vi "Continuous SFM Test.vi"() -> ()   [LabVIEW 2015]
uses:
  Waveform VIs/FM Sweep VIs/SFM-Params.ctl
panel:
  out "Waveform Graph":dbl[](graph)
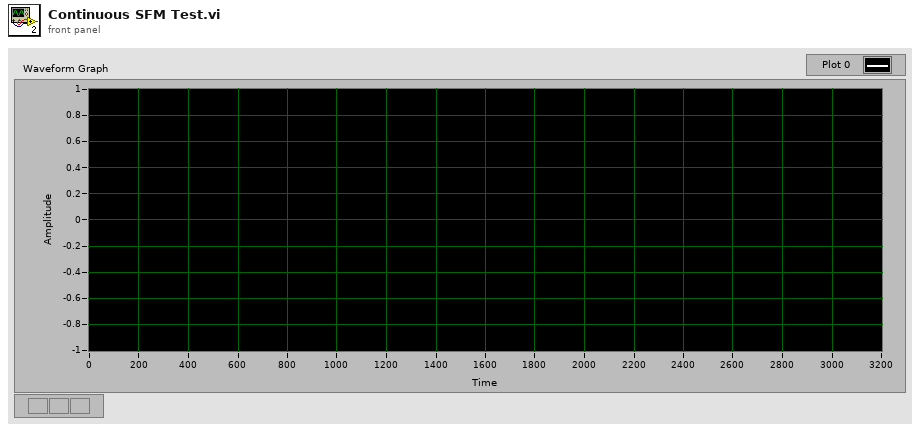
[diagram p1: front panel]
types:
  T1 = typedef "SFM-Params.ctl" = cluster{"ModArg":dbl, "MainArg":dbl, "FMod":dbl, "Fcarrier":dbl, "Fdepth":dbl}
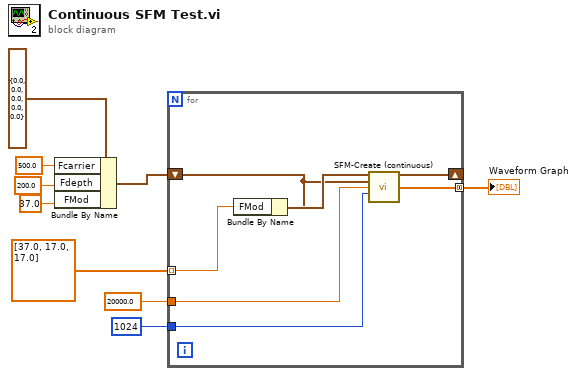
[diagram p0: block diagram]
diagram:
  n1 = Bundle By Name(cluster=T1 {"ModArg"=0.0, "MainArg"=0.0, "FMod"=0.0, "Fcarrier"=0.0, "Fdepth"=0.0} ("Out"), "Fcarrier"=500.0, "Fdepth"=200.0, "FMod"=37.0) -> (w4:T1)
  n2 = for {
    shift-right: [w16] -> _
    shift-left: w4 -> [w14]
    tunnel: 20000.0 -> [w11]
    tunnel: 1024 -> [w12]
    tunnel: [w13] -> w1 mode=concatenating
    tunnel: dbl[] [37.0, 17.0, 17.0] -> [w10] mode=indexing
    n3 = Bundle By Name(cluster=w14, "FMod"=w10) -> (w15:T1)
    n4 = call "SFM-Create (continuous).vi"("New"=w15, "Old"=w14, "Fs (Hz)"=w11, "Npts"=w12) -> ("Out"=w16:T1, "Y"=w13:dbl[])  [unwired: 10 in]
  }
  "Waveform Graph" <- w1
